vi "Push_Error.vi"(8 "error in (no error)":errorcluster, 9 "ErrorSeverity":T1, 10 "Source":string, 11 "queue error in":refnum<queue>) -> (0 "error out":errorcluster, 3 "queue error  out":refnum<queue>)   [LabVIEW 2024, in "Error.lvlib"]
uses:
  Error.lvlib
  ErrorModel/ErrorSeverity.ctl
  ErrorModel/ErrorMessage.ctl
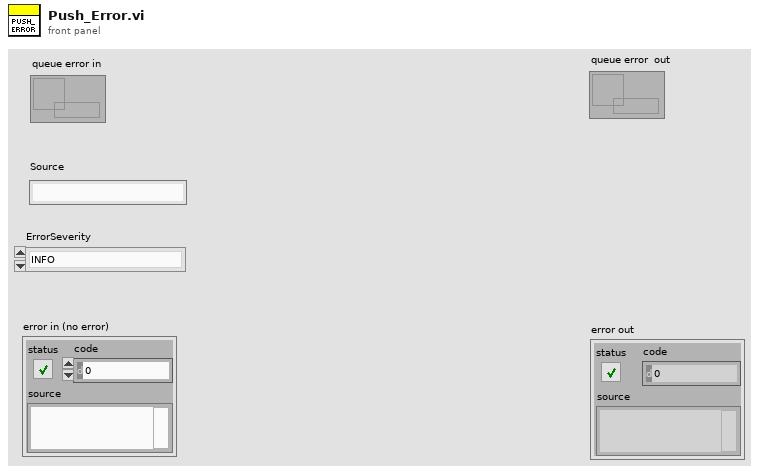
[diagram p1: front panel]
types:
  T1 = typedef "Error.lvlib/ErrorSeverity.ctl" = enum16{"INFO", "WARNING", "CRITICAL"}
  T2 = typedef "Error.lvlib/ErrorMessage.ctl" = cluster{"Time Stamp":timestamp, "Source":string, "Code":i32, "Message":string, "ErrorSeverity":T1}
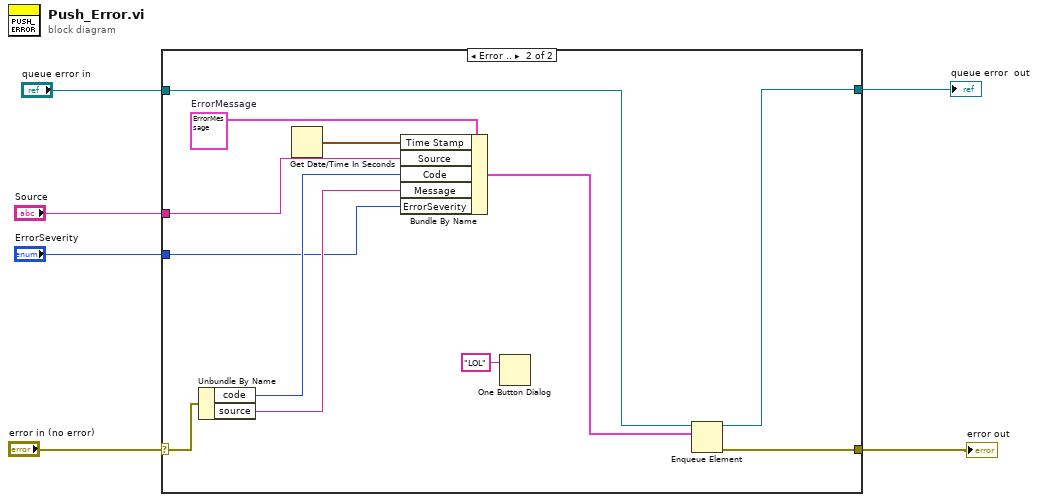
[diagram p0: block diagram]
diagram:
  n1 = case shown="Error .." "error in (no error)" {
    selector: "error in (no error)" -> [w8 w11]
    tunnel: [w8 w12] -> w5
    tunnel: "Source" -> [_ w18]
    tunnel: "ErrorSeverity" -> [_ w15]
    tunnel: "queue error in" -> [w7 w14]
    tunnel: [w7 w10] -> w1
    frame No Error {
    }
    frame Error {
      w20 = T2 {"Time Stamp"=timestamp(0 s since 1904-01-01), "Source"="", "Code"=0, "Message"="", "ErrorSeverity"=enum."INFO"}  # ErrorMessage
      n2 = Unbundle By Name(w11) -> ("code"=w17:i32, "source"=w16:string)
      n3 = Get Date/Time In Seconds() -> (seconds since 1Jan1904=w19:timestamp)
      n4 = Bundle By Name(cluster=w20, "Time Stamp"=w19, "Source"=w18, "Code"=w17, "Message"=w16, "ErrorSeverity"=w15) -> (w13:T2)
      n5 = One Button Dialog(message="LOL") -> ()  [unwired: 1 in, 1 out]
      n6 = Enqueue Element(queue=w14, element=w13) -> (queue out=w10:refnum<queue>, error out=w12:errorcluster)  [unwired: 2 in, 1 out]
    }
  }
  "error out" <- w5
  "queue error  out" <- w1
